vi "Test Return Aggregated Result for Failing Parametrized Case.vi"(11 "Test Case In":refnum<class "Parameterized Test Case Test.lvclass">) -> (0 "error out":errorcluster, 3 "Test Case Out":refnum<class "Parameterized Test Case Test.lvclass">)   [LabVIEW 2020, in "Parameterized Test Case Test.lvclass"]
uses:
  Parameterized Test Case Test.lvclass
  C:/Program Files (x86)/National Instruments/LabVIEW 2020/vi.lib/Astemes/LUnit/Test Case.lvclass
  source/Parametrized Test Case Test Double/Parametrized Test Case Test Double.lvclass
  <vilib>/Astemes/LUnit/Test Case.lvclass/Test Case.ctl
  41b79fda-963b-489b-a42a-568db35b7394.vi
  <vilib>/Astemes/LUnit/Append Pass Result.vi
  <vilib>/Astemes/LUnit/Append Fail Result.vi
  <vilib>/Astemes/LUnit/Describe Comparison.vi
  <vilib>/Astemes/LUnit/Compare Variants.vi
  <vilib>/Astemes/LUnit/Run In UI.vi
  <vilib>/Utility/error.llb/Clear Errors.vi
  <vilib>/Astemes/LUnit/Describe Variant.vi
  <vilib>/Astemes/LUnit/Test Suite.lvclass
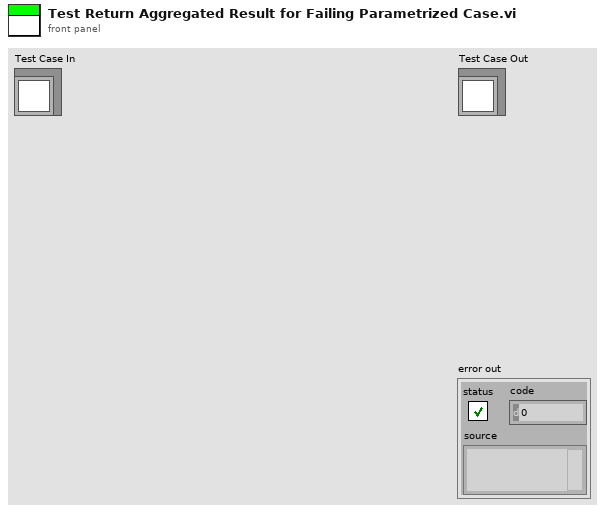
[diagram p1: front panel]
types:
  T1 = enum16{"", "Passed", "Failed", "Error", "Skipped", "Setup Error", "Broken", "Teardown Error"}
  T2 = cluster{"Name":string, "Message":string, "Description":string, "Status":enum16{"", "Passed", "Failed", "Error", "Skipped", "Setup Error", "Broken", "Teardown Error"}, "Result Type":enum16{"Test Case", "Test Suite", "Test Run", "Pass", "Fail", "Skip", "Pass if", "Fail if", "Pass if Error", "Fail if Error", "Pass if Equal", "Fail if Equal"}, "Execution Time":dbl}[]
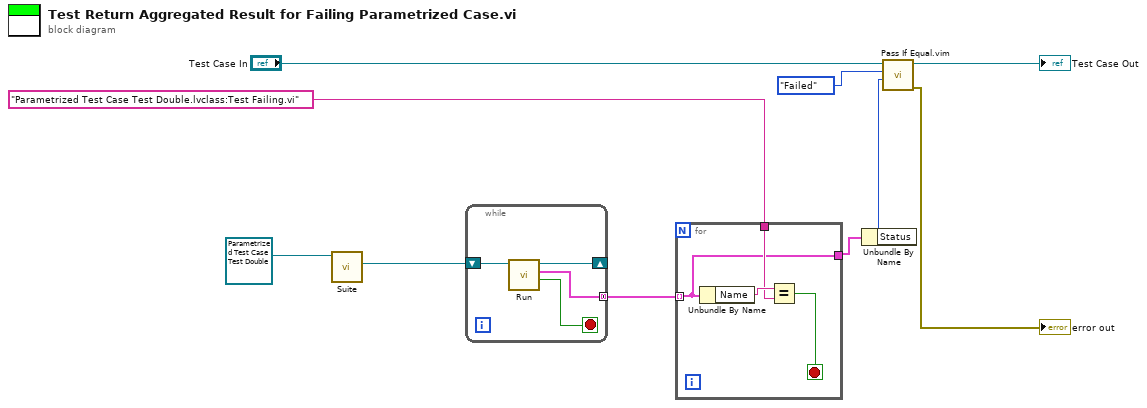
[diagram p0: block diagram]
diagram:
  n1 = call-dynamic "Suite.vi"("Parameterized Test Case In"=refnum<class "Parametrized Test Case Test Double.lvclass"> refnum ("Parametrized Test Case Test Double.lvclass")) -> ("LUnit Test Suite Out"=w6:refnum<class "Test Suite.lvclass">)  [unwired: 8 in, 2 out]
  n2 = while {
    tunnel: [w14] -> w5 mode=concatenating
    shift-right: [w12] -> _
    shift-left: w6 -> [w13]
    stop <- w11 stop-if-true
    n3 = call-dynamic "Run.vi"("LUnit Test Suite In"=w13) -> ("Done?"=w11:bool, "Results"=w14:T2, "LUnit Test Suite In 2"=w12:refnum<class "Test Suite.lvclass">)  [unwired: 7 in, 1 out]
  }
  n4 = for {
    tunnel: w5 -> [w15] mode=indexing
    tunnel: "Parametrized Test Case Test Double.lvclass:Test Failing.vi" ("String") -> [w17]
    tunnel: [w15] -> w2
    stop <- w16 stop-if-true
    n5 = Unbundle By Name(w15) -> ("Name"=w18:string)
    n6 = Equal?(x=w18, y=w17) -> (x = y?=w16:bool)
  }
  n7 = Unbundle By Name(w2) -> ("Status"=w1:T1)
  n8 = call "Pass If Equal.vim"("Actual"=w1, "Expected"=T1."Failed" ("Status"), "LUnit Test Case In"="Test Case In") -> ("error out"=→"error out":errorcluster, "LUnit Test Case Out"=→"Test Case Out":refnum<class "Parameterized Test Case Test.lvclass">)  [unwired: 7 in]
